vi "HandleError.vi"(5 "LabVIEWObjectIn":refnum<class>, 7 "MethodDataOutput":refnum<class>, 8 "ErrorIn":errorcluster, 9 "VICallError":errorcluster, 10 "CommandVI":string) -> (0 "ErrorOut":errorcluster, 3 "YActor out":refnum<class>)   [LabVIEW 2021, in "YActor.lvclass"]
uses:
  YActor.lvclass
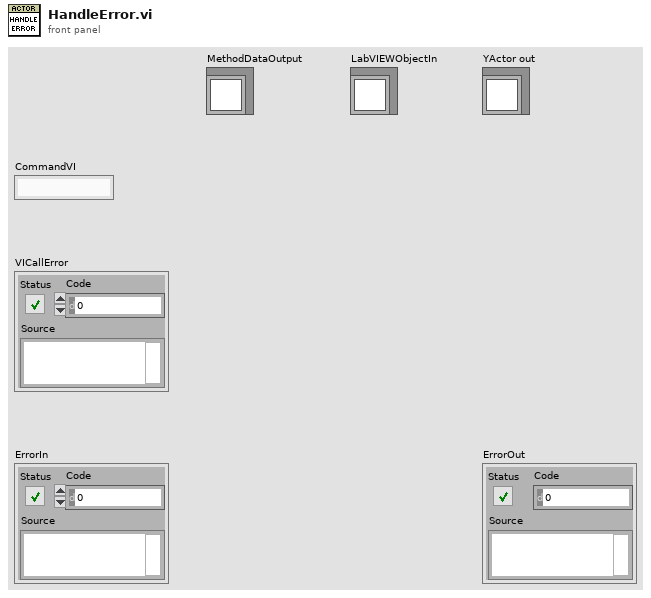
[diagram p1: front panel]
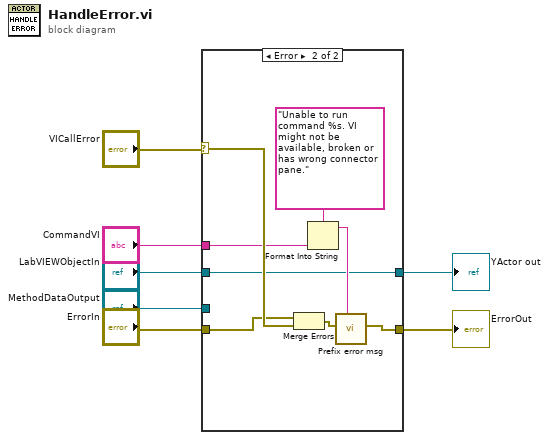
[diagram p0: block diagram]
diagram:
  n1 = case shown="Error" "VICallError" {
    selector: "VICallError" -> [_ w16]
    tunnel: "CommandVI" -> [_ w13]
    tunnel: [w9 w17] -> w5
    tunnel: "ErrorIn" -> [w9 w14]
    tunnel: "MethodDataOutput" -> [w8 _]
    tunnel: "LabVIEWObjectIn" -> [_ w10]
    tunnel: [w8 w10] -> w1
    frame No Error {
    }
    frame Error {
      n2 = Merge Errors(w14, w16) -> (w15:errorcluster)
      n3 = Format Into String(format string="Unable to run command %s. VI might not be available, broken or has wrong connector pane.", w13) -> (resulting string=w12:string)  [unwired: 2 in, 1 out]
      n4 = call "Prefix error msg.vi"("Prefix message"=w12, "error in (no error)"=w15) -> ("error out"=w17:errorcluster)  [unwired: 9 in]
    }
  }
  "ErrorOut" <- w5
  "YActor out" <- w1
